vi "getRef.vi"(8 "error in (no error)":errorcluster) -> (0 "error out":errorcluster, 2 "File Controller_ref":refnum<class "File Controller.lvclass">)   [LabVIEW 2015, in "File Controller.lvclass"]
uses:
  File Controller.lvclass
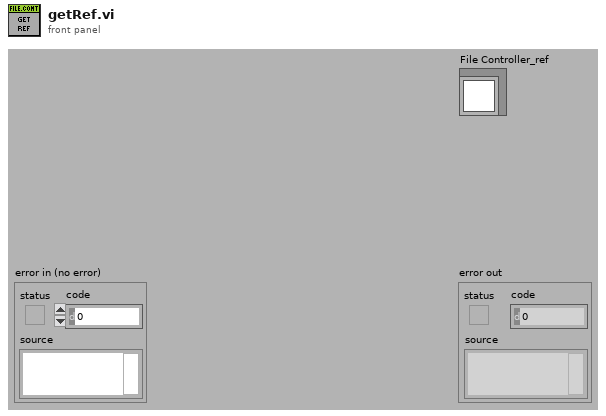
[diagram p1: front panel]
types:
  T1 = typedef "File Controller.lvclass/ClassAttributesRef.ctl" = refnum<data-value>
  T2 = typedef "File Controller.lvclass/ClassAttributes.ctl" = cluster{"Dummy":bool, "File Controller_ref":refnum<class "File Controller.lvclass">}
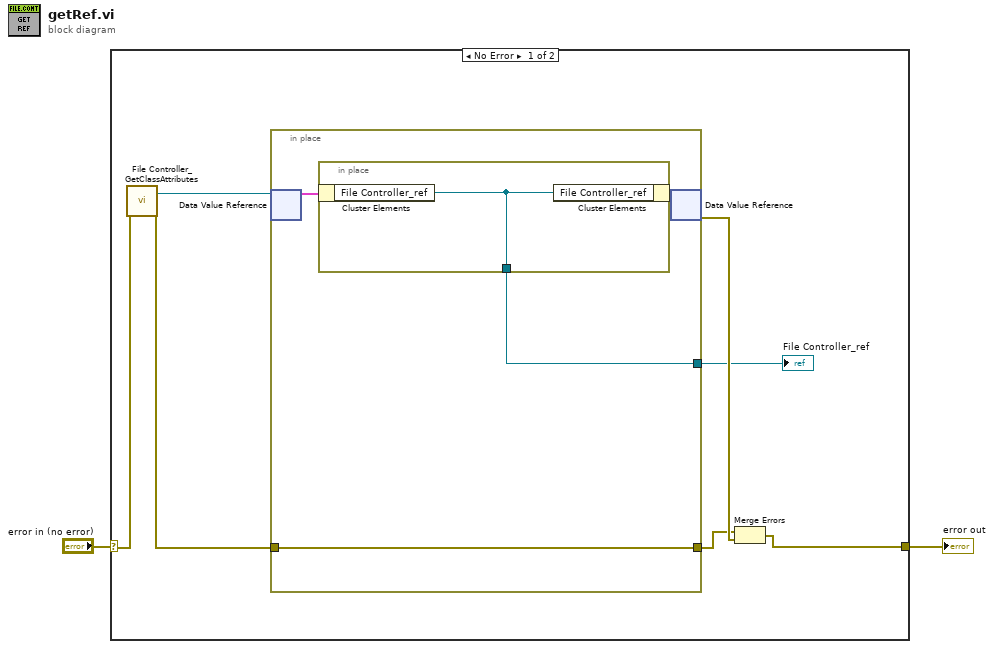
[diagram p0: block diagram]
diagram:
  n1 = case shown="No Error" "error in (no error)" {
    selector: "error in (no error)" -> [w6 w15]
    tunnel: [w9 w15] -> w1
    frame No Error {
      n2 = call "File Controller_GetClassAttributes.vi"("error in (no error)"=w6) -> ("class attributes ref"=w4:T1, "error out"=w5:errorcluster)  [unwired: 15 in, 2 out]
      n3 = in-place {
        in-place-border: w5 -> [w11]
        in-place-border: [w11] -> w7
        in-place-border: [w10] -> w3
        n4 = in-place-dvr #1(w4) -> (w12:T2)  [unwired: 1 out]
        n5 = in-place {
          in-place-border: [w14] -> w10
          n6 = in-place-cluster #2(w12) -> ("File Controller_ref"=w14:refnum<class "File Controller.lvclass">)
          n7 = in-place-cluster #2("File Controller_ref"=w14) -> (w13:T2)
        }
        n8 = in-place-dvr #1(w13) -> (w8:errorcluster)  [unwired: 1 out]
      }
      "File Controller_ref" <- w3
      n9 = Merge Errors(w7, w8) -> (w9:errorcluster)
    }
    frame Error {
    }
  }
  "error out" <- w1
